vi "main.vi"() -> ()   [LabVIEW 2016]
uses:
  <vilib>/Instr/_visa.llb/VISA Configure Serial Port (Instr).vi
panel:
  in  "Milliseconds to wait":u32
  out "LED":bool
  out "Temperatura":dbl
  in  "Set-point":i32
  out "Grafica temperatura":i32(graph)
  in  "STOP":bool
  in  "VISA resource name":refnum<visa-resource-name>
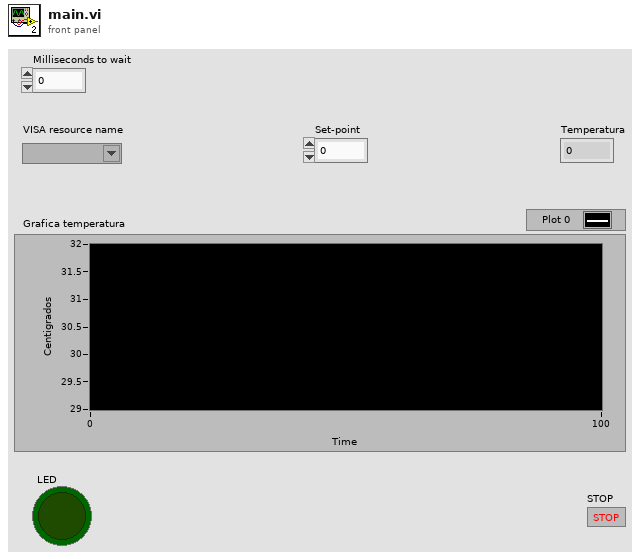
[diagram p1: front panel]
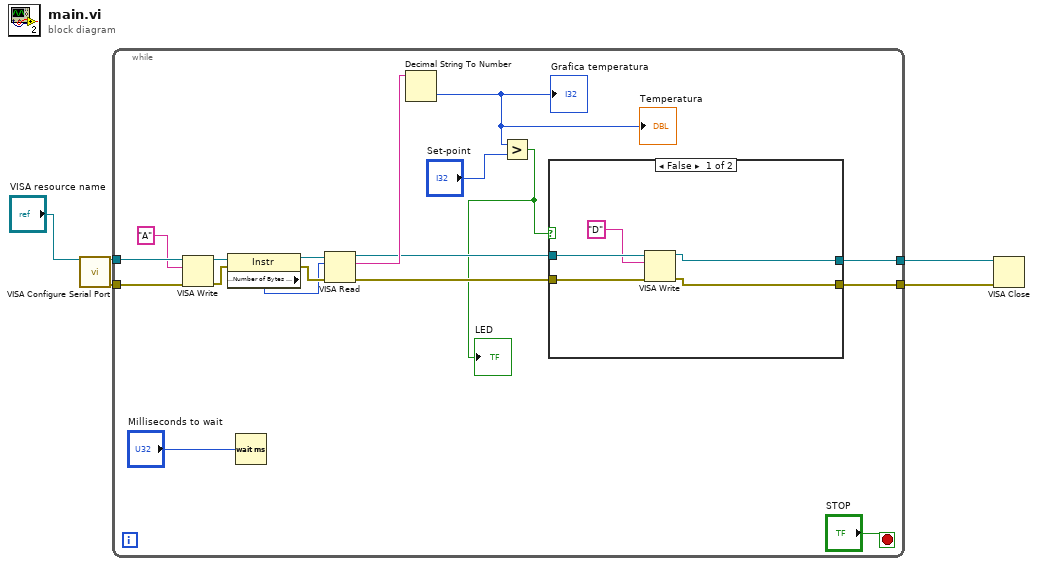
[diagram p0: block diagram]
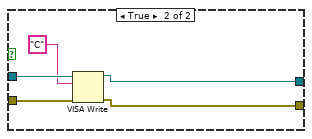
[diagram p2: hidden frame]
diagram:
  n1 = call-poly "VISA Configure Serial Port"("VISA resource name"="VISA resource name") -> ("VISA resource name out"=w5:refnum<visa-resource-name>, "error out"=w4:errorcluster)  [unwired: 13 in]
  n2 = while {
    tunnel: w5 -> [w22]
    tunnel: w4 -> [w21]
    tunnel: [w10] -> w2
    tunnel: [w9] -> w1
    stop <- "STOP" stop-if-true
    n3 = VISA Write(VISA resource name=w22, write buffer="A", error in (no error)=w21) -> (VISA resource name out=w20:refnum<visa-resource-name>, error out=w19:errorcluster)  [unwired: 1 out]
    n4 = property class="Instr"(reference=w20, error in=w19) -> (reference out=w17:refnum<visa-resource-name>, error out=w16:errorcluster, "Serial Settings:Number of Bytes at Serial Port"=w15:u32)
    n5 = Wait (ms)(milliseconds to wait="Milliseconds to wait") -> ()  [unwired: 1 out]
    n6 = VISA Read(VISA resource name=w17, byte count=w15, error in (no error)=w16) -> (VISA resource name out=w12:refnum<visa-resource-name>, read buffer=w14:string, error out=w11:errorcluster)  [unwired: 1 out]
    n7 = Decimal String To Number(string=w14) -> (number=w8:i32)  [unwired: 2 in, 1 out]
    "Grafica temperatura" <- w8
    "Temperatura" <- w8
    n8 = Greater?(x=w8, y="Set-point") -> (0:w7:bool)
    "LED" <- w7
    n9 = case shown="False" w7 {
      tunnel: w12 -> [w28 w33]
      tunnel: w11 -> [w27 w32]
      tunnel: [w25 w30] -> w10
      tunnel: [w24 w29] -> w9
      frame False {
        n10 = VISA Write(VISA resource name=w28, write buffer="D", error in (no error)=w27) -> (VISA resource name out=w25:refnum<visa-resource-name>, error out=w24:errorcluster)  [unwired: 1 out]
      }
      frame True {
        n11 = VISA Write(VISA resource name=w33, write buffer="C", error in (no error)=w32) -> (VISA resource name out=w30:refnum<visa-resource-name>, error out=w29:errorcluster)  [unwired: 1 out]
      }
    }
  }
  n12 = VISA Close(VISA resource name=w2, error in (no error)=w1) -> ()  [unwired: 1 out]
